vi "Scale.vi"(8 "error in":errorcluster, 10 "Input":variant, 11 "Linear Scaling Strategy in":refnum<class "Linear Scaling Strategy.lvclass">) -> (0 "error out":errorcluster, 2 "Output":variant, 3 "Linear Scaling Strategy out":refnum<class "Linear Scaling Strategy.lvclass">)   [LabVIEW 2024, in "HAL.lvlib" / "Linear Scaling Strategy.lvclass"]
uses:
  Linear Scaling Strategy.lvclass
  Linear Scaling Strategy.lvclass/Linear Scaling Strategy.ctl
  <userlib>/_OpenG.lib/lvdata/lvdata.llb/openg_variant.lvlib
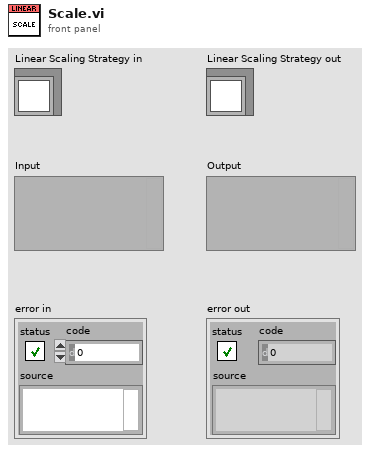
[diagram p1: front panel]
types:
  T1 = typedef "openg_variant.lvlib/Type Descriptor Enumeration__ogtk.ctl" = enum8{"<Null>", "I8", "I16", "I32", "I64", "U8", "U16", "U32", "U64", "SGL", "DBL", "EXT", "CSG", "CDB", "CXT", "0x0F", "0x10", "0x11", "0x12", "0x13", "0x14", "Enum U8", "Enum U16", "Enum U32", "Enum U64", "SGL PQ", "DBL PQ", "EXT PQ", "CSG PQ", "CDB PQ", "CXT PQ", "0x1F", "0x20", "Boolean", "0x22", "0x23", "0x24", "0x25", "0x26", "0x27", "0x28", "0x29", "0x2A", "0x2B", "0x2C", "0x2D", "0x2E", "0x2F", "String", "0x31", "Path", "Pict", "0x34", "0x35", "0x36", "DAQ", "0x38", "0x39", "0x3A", "0x3B", "0x3C", "0x3D", "0x3E", "0x3F", "Array", "0x41", "0x42", "0x43", "0x44", "0x45", "0x46", "0x47", "0x48", "0x49", "0x4A", "0x4B", "0x4C", "0x4D", "0x4E", "0x4F", "Cluster", "0x51", "0x52", "Variant", "Waveform", "0x55", "0x56", "0x57", "0x58", "0x59", "0x5A", "0x5B", "0x5C", "0x5D", "0x5E", "Fixed Point", "0x60", "0x61", "0x62", "0x63", "0x64", "0x65", "0x66", "0x67", "0x68", "0x69", "0x6A", "0x6B", "0x6C", "0x6D", "0x6E", "0x6F", "Refnum", "0x71", "0x72", "Set Collection", "Map Collection"}
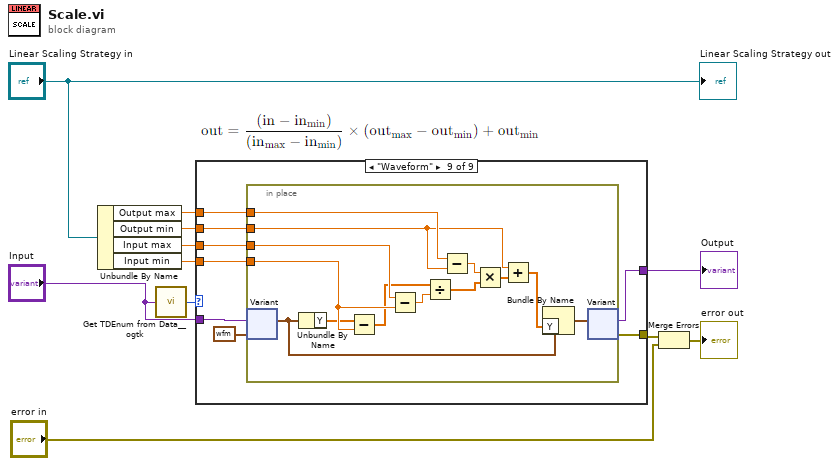
[diagram p0: block diagram]
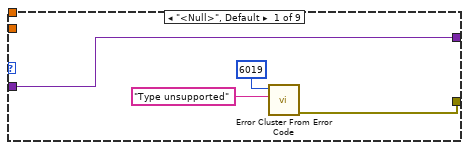
[diagram p2: hidden frame]
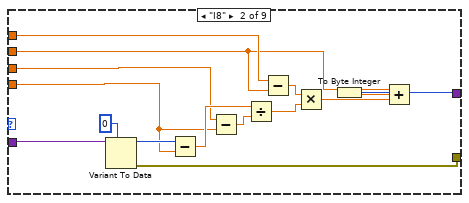
[diagram p3: hidden frame]
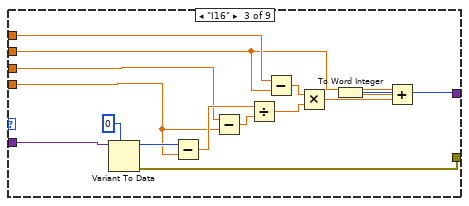
[diagram p4: hidden frame]
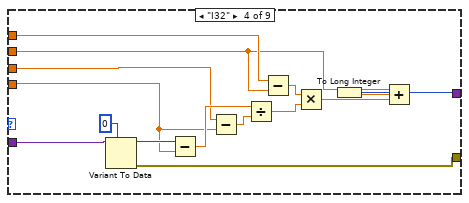
[diagram p5: hidden frame]
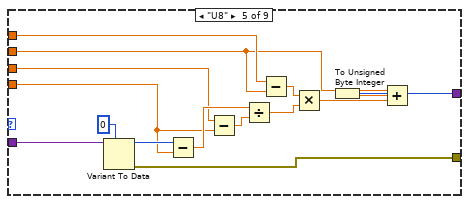
[diagram p6: hidden frame]
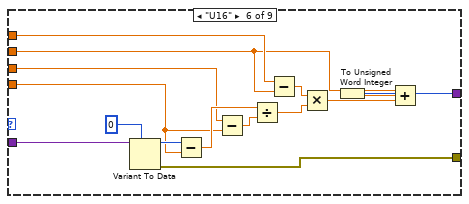
[diagram p7: hidden frame]
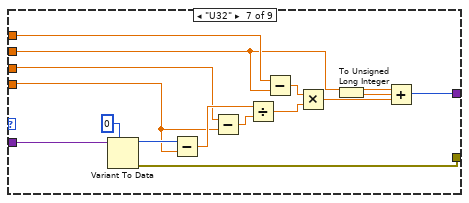
[diagram p8: hidden frame]
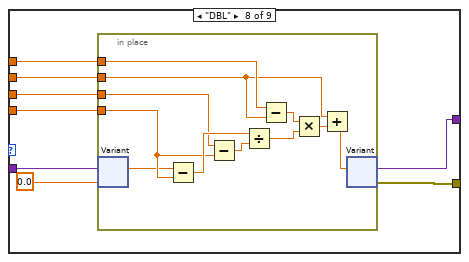
[diagram p9: hidden frame]
diagram:
  n1 = Unbundle By Name("Linear Scaling Strategy in") -> ("Output max"=w5:dbl, "Output min"=w4:dbl, "Input max"=w6:dbl, "Input min"=w7:dbl)
  n2 = call <userlib>:"Get TDEnum from Data__ogtk.vi"("Data"="Input") -> ("Type Descriptor Enumeration"=w8:T1)  [unwired: 4 in]
  n3 = case shown="\"Waveform\"" w8 {
    tunnel: "Input" -> [w15 w21 w32 w52 w63 w78 w93 w109 w132]
    tunnel: [w14 w16 w31 w46 w61 w76 w91 w106 w126] -> w3
    tunnel: [w15 w22 w37 w47 w62 w77 w92 w107 w125] -> w11
    tunnel: w7 -> [_ w17 w33 w48 w64 w79 w94 w112 w128]
    tunnel: w6 -> [_ w18 w34 w49 w65 w80 w95 w113 w129]
    tunnel: w5 -> [_ w20 w36 w51 w67 w82 w97 w111 w131]
    tunnel: w4 -> [_ w19 w35 w50 w66 w81 w96 w110 w130]
    frame "<Null>", Default {
      n4 = call <vilib>:"Error Cluster From Error Code.vi"("error message (\"\")"="Type unsupported" ("error message (\"\")"), "error code (0)"=6019) -> ("error out"=w14:errorcluster)  [unwired: 7 in]
    }
    frame "I8" {
      n5 = Variant To Data(type=i8 0, Variant=w21) -> (data=w29:i8, error out=w16:errorcluster)  [unwired: 1 in]
      n6 = Subtract(x=w29, y=w17) -> (x-y=w28:dbl)
      n7 = Subtract(x=w18, y=w17) -> (x-y=w27:dbl)
      n8 = Divide(x=w28, y=w27) -> (x/y=w25:dbl)
      n9 = Subtract(x=w20, y=w19) -> (x-y=w26:dbl)
      n10 = Multiply(x=w26, y=w25) -> (x*y=w24:dbl)
      n11 = Add(x=w19, y=w24) -> (x+y=w23:dbl)
      n12 = To Byte Integer(number=w23) -> (8bit integer=w22:i8)
    }
    frame "I16" {
      n13 = Variant To Data(type=i16 0, Variant=w32) -> (data=w44:i16, error out=w31:errorcluster)  [unwired: 1 in]
      n14 = Subtract(x=w44, y=w33) -> (x-y=w43:dbl)
      n15 = Subtract(x=w34, y=w33) -> (x-y=w42:dbl)
      n16 = Divide(x=w43, y=w42) -> (x/y=w40:dbl)
      n17 = Subtract(x=w36, y=w35) -> (x-y=w41:dbl)
      n18 = Multiply(x=w41, y=w40) -> (x*y=w39:dbl)
      n19 = Add(x=w35, y=w39) -> (x+y=w38:dbl)
      n20 = To Word Integer(number=w38) -> (16bit integer=w37:i16)
    }
    frame "I32" {
      n21 = Variant To Data(type=0, Variant=w52) -> (data=w59:i32, error out=w46:errorcluster)  [unwired: 1 in]
      n22 = Subtract(x=w59, y=w48) -> (x-y=w58:dbl)
      n23 = Subtract(x=w49, y=w48) -> (x-y=w57:dbl)
      n24 = Divide(x=w58, y=w57) -> (x/y=w55:dbl)
      n25 = Subtract(x=w51, y=w50) -> (x-y=w56:dbl)
      n26 = Multiply(x=w56, y=w55) -> (x*y=w54:dbl)
      n27 = Add(x=w50, y=w54) -> (x+y=w53:dbl)
      n28 = To Long Integer(number=w53) -> (32bit integer=w47:i32)
    }
    frame "U8" {
      n29 = Variant To Data(type=u8 0, Variant=w63) -> (data=w74:u8, error out=w61:errorcluster)  [unwired: 1 in]
      n30 = Subtract(x=w74, y=w64) -> (x-y=w73:dbl)
      n31 = Subtract(x=w65, y=w64) -> (x-y=w72:dbl)
      n32 = Divide(x=w73, y=w72) -> (x/y=w70:dbl)
      n33 = Subtract(x=w67, y=w66) -> (x-y=w71:dbl)
      n34 = Multiply(x=w71, y=w70) -> (x*y=w69:dbl)
      n35 = Add(x=w66, y=w69) -> (x+y=w68:dbl)
      n36 = To Unsigned Byte Integer(number=w68) -> (unsigned 8bit integer=w62:u8)
    }
    frame "U16" {
      n37 = Variant To Data(type=u16 0, Variant=w78) -> (data=w89:u16, error out=w76:errorcluster)  [unwired: 1 in]
      n38 = Subtract(x=w89, y=w79) -> (x-y=w88:dbl)
      n39 = Subtract(x=w80, y=w79) -> (x-y=w87:dbl)
      n40 = Divide(x=w88, y=w87) -> (x/y=w85:dbl)
      n41 = Subtract(x=w82, y=w81) -> (x-y=w86:dbl)
      n42 = Multiply(x=w86, y=w85) -> (x*y=w84:dbl)
      n43 = Add(x=w81, y=w84) -> (x+y=w83:dbl)
      n44 = To Unsigned Word Integer(number=w83) -> (unsigned 16bit integer=w77:u16)
    }
    frame "U32" {
      n45 = Variant To Data(type=u32 0, Variant=w93) -> (data=w104:u32, error out=w91:errorcluster)  [unwired: 1 in]
      n46 = Subtract(x=w104, y=w94) -> (x-y=w103:dbl)
      n47 = Subtract(x=w95, y=w94) -> (x-y=w102:dbl)
      n48 = Divide(x=w103, y=w102) -> (x/y=w100:dbl)
      n49 = Subtract(x=w97, y=w96) -> (x-y=w101:dbl)
      n50 = Multiply(x=w101, y=w100) -> (x*y=w99:dbl)
      n51 = Add(x=w96, y=w99) -> (x+y=w98:dbl)
      n52 = To Unsigned Long Integer(number=w98) -> (unsigned 32bit integer=w92:u32)
    }
    frame "DBL" {
      n53 = in-place {
        in-place-border: w113 -> [w123]
        in-place-border: w112 -> [w122]
        in-place-border: w111 -> [w120]
        in-place-border: w110 -> [w116]
        n54 = in-place-variant #1(w109, 0.0) -> (w114:dbl)  [unwired: 1 out]
        n55 = Subtract(x=w114, y=w122) -> (x-y=w124:dbl)
        n56 = Subtract(x=w123, y=w122) -> (x-y=w121:dbl)
        n57 = Divide(x=w124, y=w121) -> (x/y=w118:dbl)
        n58 = Subtract(x=w120, y=w116) -> (x-y=w119:dbl)
        n59 = Multiply(x=w119, y=w118) -> (x*y=w117:dbl)
        n60 = Add(x=w116, y=w117) -> (x+y=w115:dbl)
        n61 = in-place-variant #1(w115) -> (w107:variant, w106:errorcluster)
      }
    }
    frame "Waveform" {
      n62 = in-place {
        in-place-border: w129 -> [w145]
        in-place-border: w128 -> [w144]
        in-place-border: w131 -> [w143]
        in-place-border: w130 -> [w142]
        n63 = in-place-variant #2(w132, waveform(dbl) {"t0"=timestamp(0 s since 1904-01-01), "dt"=1.0, "Y"=[]} ("Waveform")) -> (w135:waveform(dbl))  [unwired: 1 out]
        n64 = Unbundle By Name(w135) -> ("Y"=w136:dbl[])
        n65 = Subtract(x=w136, y=w144) -> (x-y=w141:dbl[])
        n66 = Subtract(x=w145, y=w144) -> (x-y=w140:dbl)
        n67 = Divide(x=w141, y=w140) -> (x/y=w138:dbl[])
        n68 = Subtract(x=w143, y=w142) -> (x-y=w139:dbl)
        n69 = Multiply(x=w139, y=w138) -> (x*y=w137:dbl[])
        n70 = Add(x=w142, y=w137) -> (x+y=w133:dbl[])
        n71 = Bundle By Name(cluster=w135, "Y"=w133) -> (w134:waveform(dbl))
        n72 = in-place-variant #2(w134) -> (w125:variant, w126:errorcluster)
      }
    }
  }
  "Output" <- w11
  n73 = Merge Errors(w3, "error in") -> (→"error out":errorcluster)
  "Linear Scaling Strategy out" <- "Linear Scaling Strategy in"
